vi "ALTS-2015 Authentication Module.vi"(8 "Error Out":errorcluster) -> (0 "error out":errorcluster)   [LabVIEW 2013]
uses:
  Controls/ALTS-2015 Status Message Options.ctl
  Controls/ALTS-2015 User Info Cluster.ctl
  Controls/ALTS-2015 LV2GBL Restart Options.ctl
  Controls/ALTS-2015 LV2 Options.ctl
  Controls/ALTS-2015 LV2GBL Station Info Options.ctl
  Controls/ALTS-2015 LV2GBL Options.ctl
  Controls/ALTS-2015 Control Reference LV2 Options.ctl
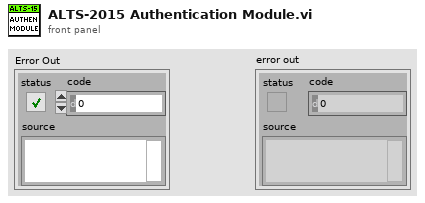
[diagram p1: front panel]
types:
  T1 = typedef "ALTS-2015 Control Reference LV2 Options.ctl" = enum16{"Set", "Get"}
  T2 = typedef "ALTS-2015 LV2GBL Restart Options.ctl" = enum16{"Get All Data", "Set Restart Notifier Ref", "Store Authentication Data"}
  T3 = typedef "ALTS-2015 LV2 Options.ctl" = enum16{"Get", "Set"}
  T4 = typedef "ALTS-2015 Status Message Options.ctl" = enum16{"Initializing...", "Enter User Login...", "Valid Serial Number...", "Invalid Serial Number...", "Start Tag Received...", "Stop Tag Received...", "UUT Clamped...", "UUT not Clamped...", "Test Running...", "Test Complete...", "Task is assigned to robot...", "Robot is working on the task...", "Robot is ready for next task...", "Writing Result to DB...", "Idle...", "Exiting..."}
  T5 = typedef "ALTS-2015 User Info Cluster.ctl" = cluster{"User 1":string, "User 2":string, "User 3":string, "User 4":string}
  T6 = typedef "ALTS-2015 Control Reference.ctl" = cluster{"User :":refnum<vi>, "Station Cluster 1":refnum<vi>, "Station Cluster 2":refnum<vi>, "Station Cluster 3":refnum<vi>, "Station Cluster 4":refnum<vi>, "Error Message":refnum<vi>, "Login/Logoff":refnum<vi>}
  T7 = typedef "ALTS-2015 LV2GBL Station Info Options.ctl" = enum16{"Init", "Read", "Read All", "Write Sensor ID", "Write  Work Order", "Write Serial Number", "Write Test Data", "Write Station Status", "Write Station Occupancy", "Write Station Test Type", "Write Rerun", "Write Load Decision", "Write Robot Action", "Clear All", "Clear Test Result"}
  T8 = enum8{"Enabled", "Disabled", "Disabled and Grayed Out"}
  T9 = typedef "ALTS-2015 LV2GBL Options.ctl" = enum16{"Read all", "Write all"}
  T10 = typedef "ALTS-2015 Station Details.ctl" = cluster{"Station Number":string, "Work Order Number":string, "Sensor Name":string, "Pressure (PSI)":string, "Flow (SCCM)":string, "Test Time ":string, "Test Result":string, "Serial Number":string, "Station Status":T11, "SW assigned UUT":bool, "Rerun Count":i32, "Test Type":i32, "Load Decision":i32, "Robot Action":T12}
  T11 = typedef "ALTS-2015 Status Ring Indicator.ctl" = u16
  T12 = typedef "ALTS-2015 Robot Actions.ctl" = enum16{"Loading...", "Unloading...", "Reruning...", "No Action"}
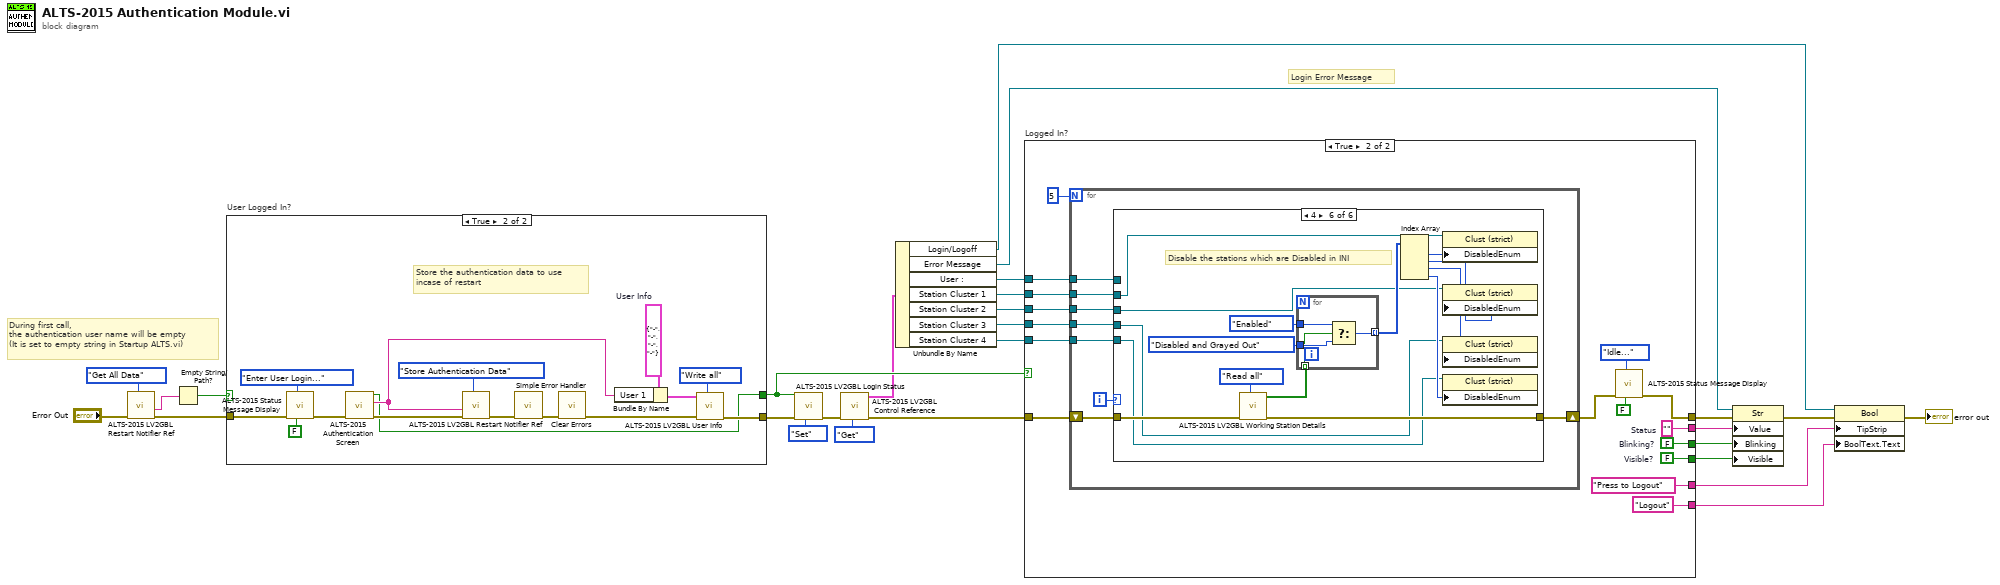
[diagram p0: block diagram]
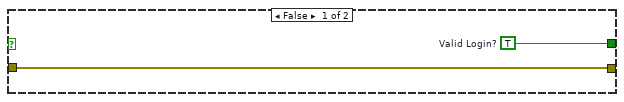
[diagram p2: hidden frame]
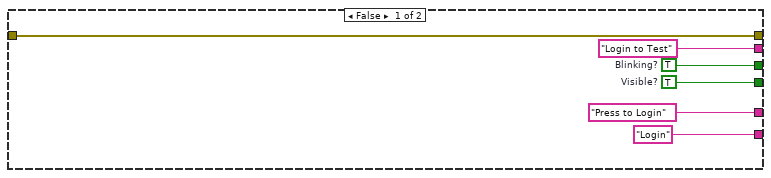
[diagram p3: hidden frame]
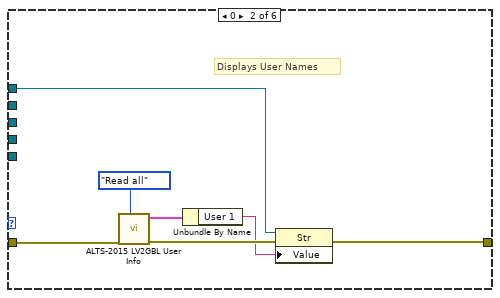
[diagram p5: hidden frame]
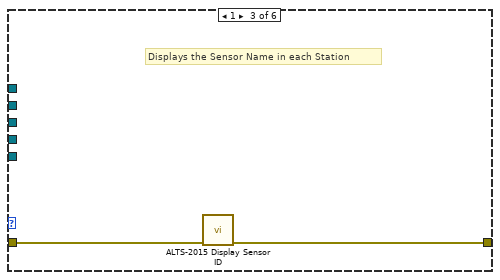
[diagram p6: hidden frame]
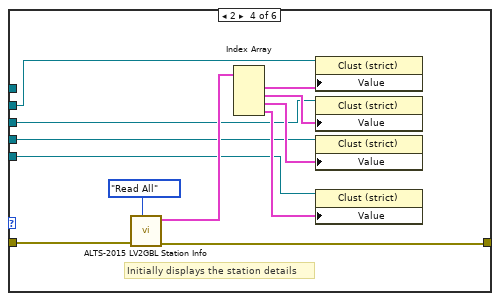
[diagram p7: hidden frame]
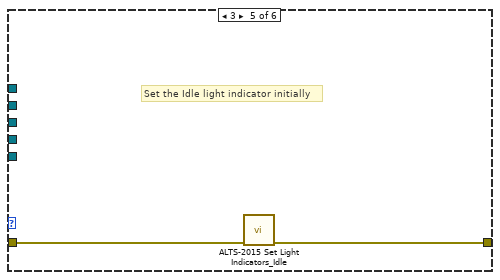
[diagram p8: hidden frame]
diagram:
  # "Login Error Message"
  # "During first call,\nthe authentication user name will be empty\n(It is set to empty string in Startup ALTS.vi)"
  n1 = call "ALTS-2015 LV2GBL Restart Notifier Ref.vi"("Options"=ALTS-2015_LV2GBL_Restart_Options."Get All Data", "Error In"="Error Out") -> ("Error Out"=w24:errorcluster, "Authenticated User Name Out"=w25:string)  [unwired: 7 in, 1 out]
  n2 = Empty String/Path?(string/path=w25) -> (empty?=w22:bool)
  n3 = case "User Logged In?" shown="True" w22 {
    tunnel: [w28 w35] -> w27
    tunnel: [w29 w34] -> w21
    tunnel: w24 -> [w28 w30]
    frame False {
      w29 = TRUE  # Valid Login?
    }
    frame True {
      w43 = T5 {"User 1"="-", "User 2"="-", "User 3"="-", "User 4"="-"}  # User Info
      # "Store the authentication data to use\nincase of restart"
      n4 = call "ALTS-2015 Status Message Display.vi"("Station Message?"=FALSE, "Status Message Options"=ALTS-2015_Status_Message_Options."Enter User Login...", "error in (no error)"=w30) -> ("error out"=w31:errorcluster)  [unwired: 7 in, 1 out]
      n5 = call "ALTS-2015 Authentication Screen.vi"("error in (no error)"=w31) -> ("error IO"=w39:errorcluster, "User Name"=w36:string, "Valid Login?"=w34:bool)  [unwired: 7 in, 1 out]
      n6 = call "ALTS-2015 LV2GBL Restart Notifier Ref.vi"("Options"=ALTS-2015_LV2GBL_Restart_Options."Store Authentication Data", "Error In"=w39, "Authenticated User Name"=w36) -> ("Error Out"=w38:errorcluster)  [unwired: 6 in, 2 out]
      n7 = call <vilib>:"Simple Error Handler.vi"("error in (no error)"=w38) -> ("error out"=w44:errorcluster)  [unwired: 4 in, 4 out]
      n8 = call <vilib>:"Clear Errors.vi"("error in (no error)"=w44) -> ("error out"=w40:errorcluster)  [unwired: 5 in, 1 out]
      n9 = Bundle By Name(cluster=w43, "User 1"=w36) -> (w42:T5)
      n10 = call "ALTS-2015 LV2GBL User Info.vi"("Options"=enum16{"Read all", "Write all"}."Write all", "error in"=w40, "User Info"=w42) -> ("error out"=w35:errorcluster)  [unwired: 7 in, 1 out]
    }
  }
  n11 = call "ALTS-2015 LV2GBL Login Status.vi"("Options"=ALTS-2015_LV2_Options."Set", "error in (no error)"=w27, "Login Status?"=w21) -> ("error out"=w18:errorcluster)  [unwired: 7 in, 1 out]
  n12 = call "ALTS-2015 LV2GBL Control Reference.vi"("LV2 Options"=ALTS-2015_Control_Reference_LV2_Options."Get", "error in"=w18) -> ("error out"=w17:errorcluster, "Control Reference_Out"=w20:T6)  [unwired: 8 in]
  n13 = Unbundle By Name(w20) -> ("Login/Logoff"=w3:refnum<vi>, "Error Message"=w10:refnum<vi>, "User :"=w16:refnum<vi>, "Station Cluster 1"=w15:refnum<vi>, "Station Cluster 2"=w14:refnum<vi>, "Station Cluster 3"=w13:refnum<vi>, "Station Cluster 4"=w12:refnum<vi>)
  n14 = case "Logged In?" shown="True" w21 {
    tunnel: w17 -> [w50 w65]
    tunnel: [w50 w51] -> w11
    tunnel: w16 -> [_ w64]
    tunnel: w15 -> [_ w63]
    tunnel: w14 -> [_ w62]
    tunnel: w13 -> [_ w61]
    tunnel: w12 -> [_ w60]
    tunnel: ["Login to Test" ("Status") w59] -> w9
    tunnel: [w48 w58] -> w8
    tunnel: [w47 w57] -> w7
    tunnel: ["Press to Login" ("Tip Strip") "Press to Logout" ("Tip Strip")] -> w2
    tunnel: ["Login" ("Boolean Text.Text") "Logout" ("Boolean Text.Text")] -> w1
    frame False {
      w47 = TRUE  # Visible?
      w48 = TRUE  # Blinking?
    }
    frame True {
      w57 = FALSE  # Visible?
      w58 = FALSE  # Blinking?
      w59 = ""  # Status
      n15 = for {
        N: 5 -> [_]
        shift-right: [w73] -> w52
        shift-left: w65 -> [w72]
        tunnel: w64 -> [w71]
        tunnel: w63 -> [w70]
        tunnel: w62 -> [w69]
        tunnel: w61 -> [w68]
        tunnel: w60 -> [w67]
        i -> [w74]
        n16 = case shown="4" w74 {
          tunnel: [w75 w77 w83 w89 w97 w107] -> w73
          tunnel: w72 -> [w75 w80 w84 w90 w98 w108]
          tunnel: w71 -> [_ w79 _ _ _ _]
          tunnel: w70 -> [_ _ _ w88 _ w102]
          tunnel: w69 -> [_ _ _ w87 _ w101]
          tunnel: w68 -> [_ _ _ w86 _ w100]
          tunnel: w67 -> [_ _ _ w85 _ w99]
          frame -1, Default {
          }
          frame 0 {
            # "Displays User Names"
            n17 = call "ALTS-2015 LV2GBL User Info.vi"("Options"=enum16{"Read all", "Write all"}."Read all", "error in"=w80) -> ("error out"=w78:errorcluster, "User Info Out"=w81:T5)  [unwired: 8 in]
            n18 = Unbundle By Name(w81) -> ("User 1"=w76:string)
            n19 = property class="Str"(reference=w79, error in=w78, "Value"=w76) -> (error out=w77:errorcluster)  [unwired: 1 out]
          }
          frame 1 {
            # "Displays the Sensor Name in each Station"
            n20 = call "ALTS-2015 Display Sensor ID.vi"("error in (no error)"=w84) -> ("error out"=w83:errorcluster)  [unwired: 10 in]
          }
          frame 2 {
            # "Initially displays the station details"
            n21 = call "ALTS-2015 LV2GBL Station Info.vi"("Options"=ALTS-2015_LV2GBL_Station_Info_Options."Read All", "error in"=w90) -> ("error out"=w89:errorcluster, "Station Info Array"=w92:T10[])  [unwired: 7 in, 1 out]
            n22 = Index Array(array=w92) -> (element #1=w93:T10, element #2=w94:T10, element #3=w95:T10, element #4=w96:T10)  [unwired: 4 in]
            n23 = property on="Property Node" class="Clust (strict)"(reference=w88, "Value"=w93) -> ()  [unwired: 1 in, 2 out]
            n24 = property on="Property Node" class="Clust (strict)"(reference=w87, "Value"=w94) -> ()  [unwired: 1 in, 2 out]
            n25 = property on="Property Node" class="Clust (strict)"(reference=w86, "Value"=w95) -> ()  [unwired: 1 in, 2 out]
            n26 = property on="Property Node" class="Clust (strict)"(reference=w85, "Value"=w96) -> ()  [unwired: 1 in, 2 out]
          }
          frame 3 {
            # "Set the Idle light indicator initially"
            n27 = call "ALTS-2015 Set Light Indicators_Idle.vi"("error in (no error)"=w98) -> ("error out"=w97:errorcluster)  [unwired: 10 in]
          }
          frame 4 {
            # "Disable the stations which are Disabled in INI"
            n28 = call "ALTS-2015 LV2GBL Working Station Details.vi"("Options"=ALTS-2015_LV2GBL_Options."Read all", "error in"=w108) -> ("error out"=w107:errorcluster, "Station  Enable Array"=w104:bool[])  [unwired: 8 in]
            n29 = for {
              tunnel: T8."Enabled" ("Disabled") -> [w117]
              tunnel: T8."Disabled and Grayed Out" ("Disabled") -> [w116]
              tunnel: w104 -> [w115] mode=indexing
              tunnel: [w114] -> w103 mode=indexing
              n30 = Select(t=w117, s=w115, f=w116) -> (s? t:f=w114:T8)
            }
            n31 = Index Array(array=w103) -> (element #1=w110:T8, element #2=w111:T8, element #3=w112:T8, element #4=w113:T8)  [unwired: 4 in]
            n32 = property on="Property Node" class="Clust (strict)"(reference=w102, "DisabledEnum"=w110) -> ()  [unwired: 1 in, 2 out]
            n33 = property on="Property Node" class="Clust (strict)"(reference=w101, "DisabledEnum"=w111) -> ()  [unwired: 1 in, 2 out]
            n34 = property on="Property Node" class="Clust (strict)"(reference=w100, "DisabledEnum"=w112) -> ()  [unwired: 1 in, 2 out]
            n35 = property on="Property Node" class="Clust (strict)"(reference=w99, "DisabledEnum"=w113) -> ()  [unwired: 1 in, 2 out]
          }
        }
      }
      n36 = call "ALTS-2015 Status Message Display.vi"("Station Message?"=FALSE, "Status Message Options"=ALTS-2015_Status_Message_Options."Idle...", "error in (no error)"=w52) -> ("error out"=w51:errorcluster)  [unwired: 7 in, 1 out]
    }
  }
  n37 = property class="Str"(reference=w10, error in=w11, "Value"=w9, "Blinking"=w8, "Visible"=w7) -> (error out=w5:errorcluster)  [unwired: 1 out]
  n38 = property class="Bool"(reference=w3, error in=w5, "TipStrip"=w2, "BoolText.Text"=w1) -> (error out=→"error out":errorcluster)  [unwired: 1 out]
